vi "Pockels-Make sequence array length even.vi"(11 "Single line AO sequence in":dbl[](array[numeric])) -> (3 "Single line AO sequence out":dbl[](array[numeric]))   [LabVIEW 2013]
uses:
  <vilib>/GPower/Comparison/Library/IsOdd/IsOddI32.vi
  <vilib>/GPower/Comparison/GPComparison.lvlib
panel:
  out "Output length":i32
  out "Input length":i32
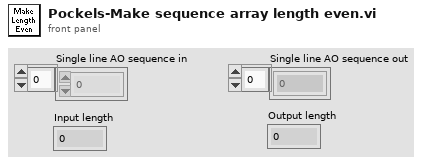
[diagram p1: front panel]
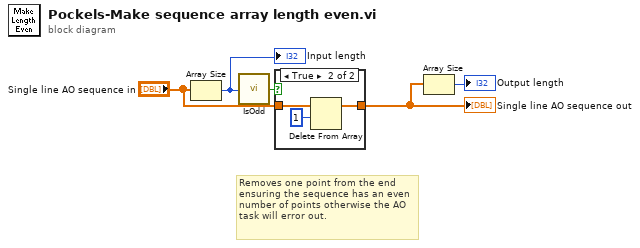
[diagram p0: block diagram]
diagram:
  # "Removes one point from the end ensuring the sequence has an even number of points otherwise the AO task will error out."
  n1 = Array Size(array="Single line AO sequence in") -> (size(s)=w1:i32)
  "Input length" <- w1
  n2 = call-poly <vilib>:"IsOdd.vi"("x"=w1) -> ("Odd?"=w4:bool)  [unwired: 4 in]
  n3 = case shown="True" w4 {
    tunnel: "Single line AO sequence in" -> [w6 w9]
    tunnel: [w6 w8] -> w2
    frame False {
    }
    frame True {
      n4 = Delete From Array(array=w9, length=1) -> (array with subset deleted=w8:dbl[])  [unwired: 1 in, 1 out]
    }
  }
  "Single line AO sequence out" <- w2
  n5 = Array Size(array=w2) -> (size(s)=→"Output length":i32)
